vi "GEOM_chk_override_format.vi"(9 "arguments":string[](array[string]), 10 "switches":string[](array[string])) -> (1 "format OK":bool, 2 "format out":string)   [LabVIEW 2016]
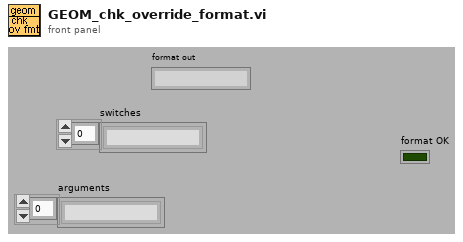
[diagram p1: front panel]
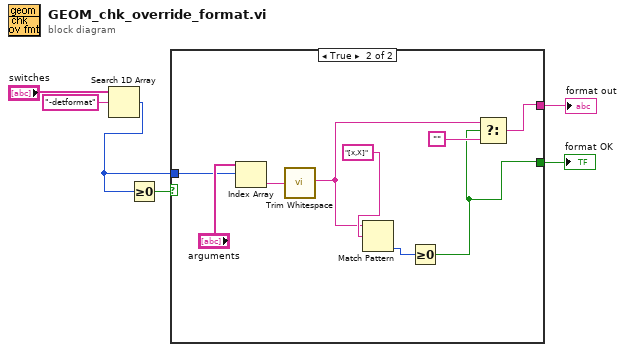
[diagram p0: block diagram]
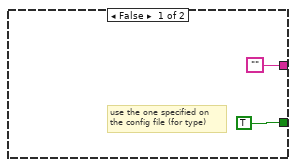
[diagram p2: hidden frame]
diagram:
  n1 = Search 1D Array(1D array="switches", element="-detformat") -> (index of element=w2:i32)  [unwired: 1 out]
  n2 = Greater Or Equal To 0?(x=w2) -> (x >= 0?=w4:bool)
  n3 = case shown="True" w4 {
    tunnel: ["" w13] -> w3
    tunnel: w2 -> [_ w16]
    tunnel: [TRUE ("format OK") w9] -> w1
    frame False {
      # "use the one specified on\nthe config file (for type)"
    }
    frame True {
      n4 = Index Array(array="arguments", index=w16) -> (element=w15:string)
      n5 = call <vilib>:"Trim Whitespace.vi"("string"=w15) -> ("trimmed string"=w11:string)  [unwired: 1 in]
      n6 = Match Pattern(string=w11, regular expression="[x,X]" ("separator")) -> (offset past match=w10:i32)  [unwired: 4 out]
      n7 = Greater Or Equal To 0?(x=w10) -> (x >= 0?=w9:bool)
      n8 = Select(t=w11, s=w9, f="") -> (s? t:f=w13:string)
    }
  }
  "format out" <- w3
  "format OK" <- w1
